vi "DMM 7_5 Digit Histogram.vi"() -> ()   [LabVIEW 2019]
uses:
  OCVResults.ctl
  <vilib>/Analysis/NI_AALBase.lvlib
  <vilib>/gmath/NI_Gmath.lvlib
panel:
  in  "Measurements (Volts) ch4 2":dbl[](array[numeric])=[3.486017932336771, 3.486017307834901, 3.486017600737179, 3.486017977248404, 3.4860177403183688, 3.4860179150120914, 3.4860177036838285, 3.4860178309889314, 3.4860177531972822, 3.486017977754826, 3.4860179330089647, 3.48601814510014, 3.486018147033395, 3.4860177431187243, 3.4860177797011875, 3.486017997042972, 3.486018038037714, 3.486017878191467, 3.486018126596086, 3.486017769724553, 3.486017992593923, 3.4860184321660705, 3.486017864938252, 3.486017411838484, 3.4860179876723802, 3.486017959684013, 3.4860179763899417, 3.4860178187665127, 3.4860181827150996, 3.486018245194682, 3.4860180098625495, 3.486017797221756, 3.4860181423306345, 3.4860176881665175, 3.486018084873098, 3.486017671108277, 3.4860178318523425, 3.4860176788045503, 3.4860177962648726, 3.4860176851712743, 3.486017790116506, 3.4860177670877572, 3.486018012605684, 3.4860178934400214, 3.486018329992307, 3.4860180981146773, 3.4860180096557576, 3.486017938785145, 3.4860183230428614, 3.4860178747798787, 3.486017814818513, 3.4860179148088757, 3.4860181999824875, 3.486017785602333, 3.486017829577085, 3.4860180105835474, 3.4860174289366563, 3.486017644862929, 3.4860178994496565, 3.4860179954448096, 3.48601793934282, 3.4860179746921376, 3.486018026188553, 3.4860175892288225, 3.4860180347614023, 3.4860181103873873, 3.4860178832560527, 3.4860180410479487, 3.486018032763997, 3.486018622537674, 3.4860181548045874, 3.486017530224023, 3.486017947248753, 3.486018043066002, 3.48601811908244, 3.4860179760940153, 3.486018418334813, 3.4860178982991576, 3.4860182376122486, 3.486017987488014, 3.486017961989586, 3.486017839712657, 3.486018154426059, 3.4860182654538283, 3.486018068682808, 3.486017939355624, 3.486018112168974, 3.486018021643548, 3.4860181301969235, 3.4860181388493037, 3.486018377605749, 3.4860181136864066, 3.4860176318841773, 3.4860180166697994, 3.4860177217403545, 3.4860181410713804, 3.4860178522251486, 3.486017813379955, 3.486018026525973, 3.4860178772425607] format="%#_9g"
  out "Results":T1={"V ch0 Array"=[2.6402355104591723e-06, 3.2050422226470716e-06, 3.2738385547093894e-06, 3.0004056082675545e-06, 3.190429018678622e-06, 3.265655292871135e-06, 3.4283206777974678e-06], "V ch1 Array"=[3.579181433209794e-06, 3.538102305000126e-06, 3.3674070559982216e-06, 3.2951997357567907e-06, 3.0614196043446336e-06, 3.247982674682344e-06, 3.4582756481500834e-06], "V ch2 Array"=[2.636942617106564e-06, 2.444215695573972e-06, 2.3600385872845126e-06, 2.3785120159418297e-06, 2.39158079459529e-06, 2.5415574149365358e-06, 2.629696833600491e-06], "V ch3 Array"=[4.29015971742814e-06, 4.582682915243894e-06, 4.199947801068903e-06, 4.210565880465411e-06, 4.1249236933492e-06, 4.3283146693326225e-06], "V ch4 Array"=[3.2068632920738282e-06, 3.2352868353418705e-06, 3.218523090660476e-06, 3.1985005992771743e-06, 3.2252632419667723e-06, 3.3472279144313767e-06], "Elapsed Time (ms)"=11164, "DMM Fault Array"=[]}
  in  "Measurements (Volts) ch4":dbl[](array[numeric])=[3.486017932336771, 3.486017307834901, 3.486017600737179, 3.486017977248404, 3.4860177403183688, 3.4860179150120914, 3.4860177036838285, 3.4860178309889314, 3.4860177531972822, 3.486017977754826, 3.4860179330089647, 3.48601814510014, 3.486018147033395, 3.4860177431187243, 3.4860177797011875, 3.486017997042972, 3.486018038037714, 3.486017878191467, 3.486018126596086, 3.486017769724553, 3.486017992593923, 3.4860184321660705, 3.486017864938252, 3.486017411838484, 3.4860179876723802, 3.486017959684013, 3.4860179763899417, 3.4860178187665127, 3.4860181827150996, 3.486018245194682, 3.4860180098625495, 3.486017797221756, 3.4860181423306345, 3.4860176881665175, 3.486018084873098, 3.486017671108277, 3.4860178318523425, 3.4860176788045503, 3.4860177962648726, 3.4860176851712743, 3.486017790116506, 3.4860177670877572, 3.486018012605684, 3.4860178934400214, 3.486018329992307, 3.4860180981146773, 3.4860180096557576, 3.486017938785145, 3.4860183230428614, 3.4860178747798787, 3.486017814818513, 3.4860179148088757, 3.4860181999824875, 3.486017785602333, 3.486017829577085, 3.4860180105835474, 3.4860174289366563, 3.486017644862929, 3.4860178994496565, 3.4860179954448096, 3.48601793934282, 3.4860179746921376, 3.486018026188553, 3.4860175892288225, 3.4860180347614023, 3.4860181103873873, 3.4860178832560527, 3.4860180410479487, 3.486018032763997, 3.486018622537674, 3.4860181548045874, 3.486017530224023, 3.486017947248753, 3.486018043066002, 3.48601811908244, 3.4860179760940153, 3.486018418334813, 3.4860178982991576, 3.4860182376122486, 3.486017987488014, 3.486017961989586, 3.486017839712657, 3.486018154426059, 3.4860182654538283, 3.486018068682808, 3.486017939355624, 3.486018112168974, 3.486018021643548, 3.4860181301969235, 3.4860181388493037, 3.486018377605749, 3.4860181136864066, 3.4860176318841773, 3.4860180166697994, 3.4860177217403545, 3.4860181410713804, 3.4860178522251486, 3.486017813379955, 3.486018026525973, 3.4860178772425607] format="%#_9g"
  in  "Measurements (Volts) ch3":dbl[](array[numeric])=[3.486017932336771, 3.486017307834901, 3.486017600737179, 3.486017977248404, 3.4860177403183688, 3.4860179150120914, 3.4860177036838285, 3.4860178309889314, 3.4860177531972822, 3.486017977754826, 3.4860179330089647, 3.48601814510014, 3.486018147033395, 3.4860177431187243, 3.4860177797011875, 3.486017997042972, 3.486018038037714, 3.486017878191467, 3.486018126596086, 3.486017769724553, 3.486017992593923, 3.4860184321660705, 3.486017864938252, 3.486017411838484, 3.4860179876723802, 3.486017959684013, 3.4860179763899417, 3.4860178187665127, 3.4860181827150996, 3.486018245194682, 3.4860180098625495, 3.486017797221756, 3.4860181423306345, 3.4860176881665175, 3.486018084873098, 3.486017671108277, 3.4860178318523425, 3.4860176788045503, 3.4860177962648726, 3.4860176851712743, 3.486017790116506, 3.4860177670877572, 3.486018012605684, 3.4860178934400214, 3.486018329992307, 3.4860180981146773, 3.4860180096557576, 3.486017938785145, 3.4860183230428614, 3.4860178747798787, 3.486017814818513, 3.4860179148088757, 3.4860181999824875, 3.486017785602333, 3.486017829577085, 3.4860180105835474, 3.4860174289366563, 3.486017644862929, 3.4860178994496565, 3.4860179954448096, 3.48601793934282, 3.4860179746921376, 3.486018026188553, 3.4860175892288225, 3.4860180347614023, 3.4860181103873873, 3.4860178832560527, 3.4860180410479487, 3.486018032763997, 3.486018622537674, 3.4860181548045874, 3.486017530224023, 3.486017947248753, 3.486018043066002, 3.48601811908244, 3.4860179760940153, 3.486018418334813, 3.4860178982991576, 3.4860182376122486, 3.486017987488014, 3.486017961989586, 3.486017839712657, 3.486018154426059, 3.4860182654538283, 3.486018068682808, 3.486017939355624, 3.486018112168974, 3.486018021643548, 3.4860181301969235, 3.4860181388493037, 3.486018377605749, 3.4860181136864066, 3.4860176318841773, 3.4860180166697994, 3.4860177217403545, 3.4860181410713804, 3.4860178522251486, 3.486017813379955, 3.486018026525973, 3.4860178772425607] format="%#_9g"
  in  "Measurements (Volts) ch2":dbl[](array[numeric])=[3.486017932336771, 3.486017307834901, 3.486017600737179, 3.486017977248404, 3.4860177403183688, 3.4860179150120914, 3.4860177036838285, 3.4860178309889314, 3.4860177531972822, 3.486017977754826, 3.4860179330089647, 3.48601814510014, 3.486018147033395, 3.4860177431187243, 3.4860177797011875, 3.486017997042972, 3.486018038037714, 3.486017878191467, 3.486018126596086, 3.486017769724553, 3.486017992593923, 3.4860184321660705, 3.486017864938252, 3.486017411838484, 3.4860179876723802, 3.486017959684013, 3.4860179763899417, 3.4860178187665127, 3.4860181827150996, 3.486018245194682, 3.4860180098625495, 3.486017797221756, 3.4860181423306345, 3.4860176881665175, 3.486018084873098, 3.486017671108277, 3.4860178318523425, 3.4860176788045503, 3.4860177962648726, 3.4860176851712743, 3.486017790116506, 3.4860177670877572, 3.486018012605684, 3.4860178934400214, 3.486018329992307, 3.4860180981146773, 3.4860180096557576, 3.486017938785145, 3.4860183230428614, 3.4860178747798787, 3.486017814818513, 3.4860179148088757, 3.4860181999824875, 3.486017785602333, 3.486017829577085, 3.4860180105835474, 3.4860174289366563, 3.486017644862929, 3.4860178994496565, 3.4860179954448096, 3.48601793934282, 3.4860179746921376, 3.486018026188553, 3.4860175892288225, 3.4860180347614023, 3.4860181103873873, 3.4860178832560527, 3.4860180410479487, 3.486018032763997, 3.486018622537674, 3.4860181548045874, 3.486017530224023, 3.486017947248753, 3.486018043066002, 3.48601811908244, 3.4860179760940153, 3.486018418334813, 3.4860178982991576, 3.4860182376122486, 3.486017987488014, 3.486017961989586, 3.486017839712657, 3.486018154426059, 3.4860182654538283, 3.486018068682808, 3.486017939355624, 3.486018112168974, 3.486018021643548, 3.4860181301969235, 3.4860181388493037, 3.486018377605749, 3.4860181136864066, 3.4860176318841773, 3.4860180166697994, 3.4860177217403545, 3.4860181410713804, 3.4860178522251486, 3.486017813379955, 3.486018026525973, 3.4860178772425607] format="%#_9g"
  in  "Measurements (Volts) ch1":dbl[](array[numeric])=[3.486017932336771, 3.486017307834901, 3.486017600737179, 3.486017977248404, 3.4860177403183688, 3.4860179150120914, 3.4860177036838285, 3.4860178309889314, 3.4860177531972822, 3.486017977754826, 3.4860179330089647, 3.48601814510014, 3.486018147033395, 3.4860177431187243, 3.4860177797011875, 3.486017997042972, 3.486018038037714, 3.486017878191467, 3.486018126596086, 3.486017769724553, 3.486017992593923, 3.4860184321660705, 3.486017864938252, 3.486017411838484, 3.4860179876723802, 3.486017959684013, 3.4860179763899417, 3.4860178187665127, 3.4860181827150996, 3.486018245194682, 3.4860180098625495, 3.486017797221756, 3.4860181423306345, 3.4860176881665175, 3.486018084873098, 3.486017671108277, 3.4860178318523425, 3.4860176788045503, 3.4860177962648726, 3.4860176851712743, 3.486017790116506, 3.4860177670877572, 3.486018012605684, 3.4860178934400214, 3.486018329992307, 3.4860180981146773, 3.4860180096557576, 3.486017938785145, 3.4860183230428614, 3.4860178747798787, 3.486017814818513, 3.4860179148088757, 3.4860181999824875, 3.486017785602333, 3.486017829577085, 3.4860180105835474, 3.4860174289366563, 3.486017644862929, 3.4860178994496565, 3.4860179954448096, 3.48601793934282, 3.4860179746921376, 3.486018026188553, 3.4860175892288225, 3.4860180347614023, 3.4860181103873873, 3.4860178832560527, 3.4860180410479487, 3.486018032763997, 3.486018622537674, 3.4860181548045874, 3.486017530224023, 3.486017947248753, 3.486018043066002, 3.48601811908244, 3.4860179760940153, 3.486018418334813, 3.4860178982991576, 3.4860182376122486, 3.486017987488014, 3.486017961989586, 3.486017839712657, 3.486018154426059, 3.4860182654538283, 3.486018068682808, 3.486017939355624, 3.486018112168974, 3.486018021643548, 3.4860181301969235, 3.4860181388493037, 3.486018377605749, 3.4860181136864066, 3.4860176318841773, 3.4860180166697994, 3.4860177217403545, 3.4860181410713804, 3.4860178522251486, 3.486017813379955, 3.486018026525973, 3.4860178772425607] format="%#_9g"
  in  "Measurements (Volts) ch0":dbl[](array[numeric]) format="%#_9g"
  out "ch4 range":dbl=4.122037172130473e-07 format="%#_6p"
  out "ch4 std dev":dbl=1.1334695003754112e-07 format="%#.3p"
  out "ch4 mean":dbl=2.8507857826555935e-06 format="%#.3p"
  out "Histogram Graph ch4":T2(graph)={"X Values"=[2.6687076322194884e-06, 2.7099280039407933e-06, 2.751148375662098e-06, 2.792368747383403e-06, 2.833589119104708e-06, 2.874809490826013e-06, 2.9160298625473178e-06, 2.9572502342686227e-06, 2.9984706059899276e-06, 3.0396909777112325e-06], "Histogram: h(x)"=[1, 0, 0, 0, 2, 2, 1, 0, 0, 1]}
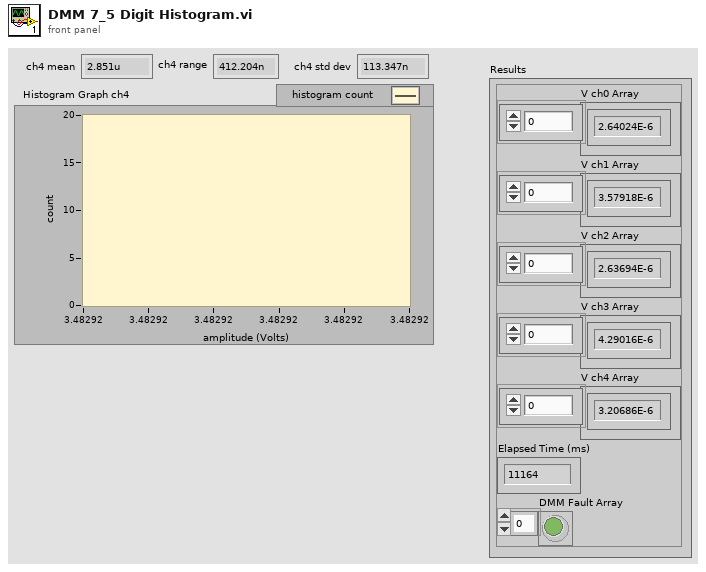
[diagram p1: front panel]
types:
  T1 = typedef "OCVResults.ctl" = cluster{"V ch0 Array":dbl[], "V ch1 Array":dbl[], "V ch2 Array":dbl[], "V ch3 Array":dbl[], "V ch4 Array":dbl[], "Elapsed Time (ms)":u32, "DMM Fault Array":bool[]}
  T2 = cluster{"X Values":dbl[], "Histogram: h(x)":i32[]}
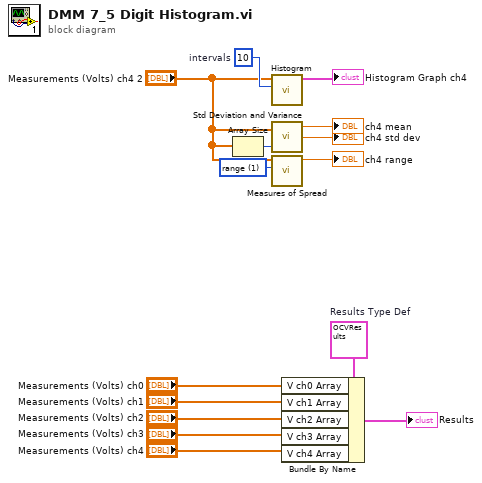
[diagram p0: block diagram]
diagram:
  w8 = T1 {"V ch0 Array"=[2.6402355104591723e-06, 3.2050422226470716e-06, 3.2738385547093894e-06, 3.0004056082675545e-06, 3.190429018678622e-06, 3.265655292871135e-06, 3.4283206777974678e-06], "V ch1 Array"=[3.579181433209794e-06, 3.538102305000126e-06, 3.3674070559982216e-06, 3.2951997357567907e-06, 3.0614196043446336e-06, 3.247982674682344e-06, 3.4582756481500834e-06], "V ch2 Array"=[2.636942617106564e-06, 2.444215695573972e-06, 2.3600385872845126e-06, 2.3785120159418297e-06, 2.39158079459529e-06, 2.5415574149365358e-06, 2.629696833600491e-06], "V ch3 Array"=[4.29015971742814e-06, 4.582682915243894e-06, 4.199947801068903e-06, 4.210565880465411e-06, 4.1249236933492e-06, 4.3283146693326225e-06], "V ch4 Array"=[3.2068632920738282e-06, 3.2352868353418705e-06, 3.218523090660476e-06, 3.1985005992771743e-06, 3.2252632419667723e-06, 3.3472279144313767e-06], "Elapsed Time (ms)"=11164, "DMM Fault Array"=[]}  # Results Type Def
  w12 = 1 items=["standard deviation", "range", "mean absolute deviation", "interquartile range"] ("type")
  w15 = 10  # intervals
  n1 = Array Size(array="Measurements (Volts) ch4 2") -> (size(s)=w13:i32)
  n2 = call <vilib>:"Histogram.vi"("intervals"=w15, "X"="Measurements (Volts) ch4 2") -> ("Histogram Graph"=→"Histogram Graph ch4":T2)  [unwired: 6 in, 3 out]
  n3 = call <vilib>:"Std Deviation and Variance.vi"("X"="Measurements (Volts) ch4 2", "Weighting (Sample)"=w13) -> ("mean"=→"ch4 mean":dbl, "standard deviation"=→"ch4 std dev":dbl)  [unwired: 1 out]
  n4 = call <vilib>:"Measures of Spread.vi"("type"=w12, "x array"="Measurements (Volts) ch4 2") -> ("spread value"=→"ch4 range":dbl)  [unwired: 8 in, 1 out]
  n5 = Bundle By Name(cluster=w8, "V ch0 Array"="Measurements (Volts) ch0", "V ch1 Array"="Measurements (Volts) ch1", "V ch2 Array"="Measurements (Volts) ch2", "V ch3 Array"="Measurements (Volts) ch3", "V ch4 Array"="Measurements (Volts) ch4") -> (→"Results":T1)
